vi "CleanUp.vi"(0 "object in":refnum<class "AdvanceTable.lvclass">, 5 "error in (no error)":errorcluster) -> (14 "object out":refnum<class "AdvanceTable.lvclass">, 19 "error out":errorcluster)   [LabVIEW 2015, in "ActorManagement.lvlib" / "AdvanceTable.lvclass"]
uses:
  AdvanceTable.lvclass
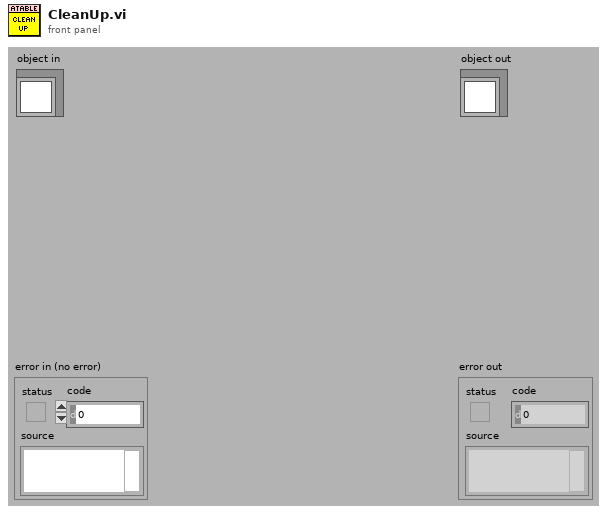
[diagram p1: front panel]
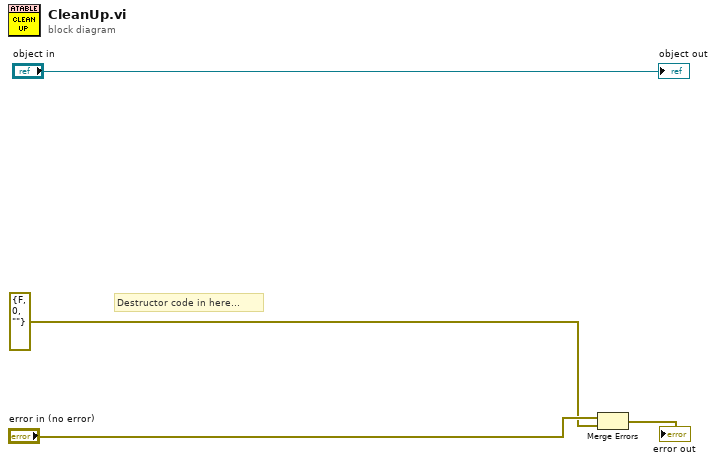
[diagram p0: block diagram]
diagram:
  # "Destructor code in here..."
  n1 = Merge Errors("error in (no error)", errorcluster {"status"=FALSE, "code"=0, "source"=""} ("error in (no error)")) -> (→"error out":errorcluster)
  "object out" <- "object in"
